vi "AgPSA _SetRef.vi"(8 "error in (no error)":errorcluster, 10 "Set External":bool, 11 "VISA resource name":refnum<visa-resource-name>) -> (0 "error out":errorcluster, 3 "VISA resource name out":refnum<visa-resource-name>)   [LabVIEW 2015]
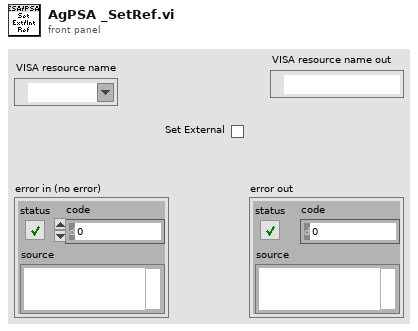
[diagram p1: front panel]
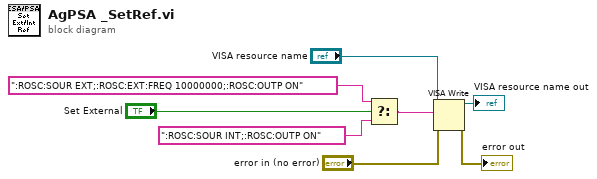
[diagram p0: block diagram]
diagram:
  n1 = Select(t=":ROSC:SOUR EXT;:ROSC:EXT:FREQ 10000000;:ROSC:OUTP ON" ("write buffer"), s="Set External", f=":ROSC:SOUR INT;:ROSC:OUTP ON" ("write buffer")) -> (s? t:f=w8:string)
  n2 = VISA Write(VISA resource name="VISA resource name", write buffer=w8, error in (no error)="error in (no error)") -> (VISA resource name out=→"VISA resource name out":refnum<visa-resource-name>, error out=→"error out":errorcluster)  [unwired: 1 out]
